vi "1 Ball Low Goal Hot.vi"(1 "Run?":bool) -> (0 "Done?":bool)   [LabVIEW 2013]
uses:
  Globals/Homes.vi
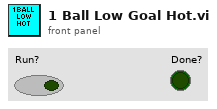
[diagram p1: front panel]
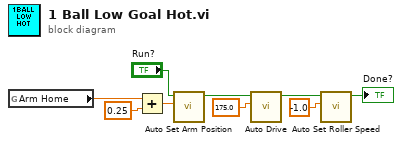
[diagram p0: block diagram]
diagram:
  n1 = global read "Homes.vi" "Arm Home"() -> (w8:dbl)
  n2 = Add(x=w8, y=0.25) -> (x+y=w7:dbl)
  n3 = call "Auto Set Arm Position.vi"("Arm Position"=w7, "Run?"="Run?") -> ("Done"=w9:bool)  [unwired: 9 in]
  n4 = call "Auto Drive.vi"("Amount"=175.0, "Run?"=w9) -> ("Done"=w1:bool)  [unwired: 9 in]
  n5 = call "Auto Set Roller Speed.vi"("Value"=-1.0, "Run?"=w1) -> ("Done"=→"Done?":bool)  [unwired: 9 in]
